vi "2D FFT and IFFT Example.vi"() -> ()   [LabVIEW 2012]
uses:
  Non-User VIs/Error Checking/View Error Log Mode Functional Global.vi
  OpenCLV x64.lvlib
panel:
  out "Labview Data":dbl[][](array[numeric])
  out "OpenCLV Data":dbl[][](array[numeric])
  out "OpenCLV Time":u32
  out "Labview Time":u32
  in  "FFT Dimension":enum16{"1D FFT", "2D FFT"}(ring)=enum."2D FFT"
  in  "Dimension":cluster{"Depth":u64, "Height":u64, "Width":u64}={"Depth"=1, "Height"=1000, "Width"=1024} {"Width" min=1; "Height" min=1; "Depth" min=1}
  # "Outputs"
  # "Inputs - Change before running"
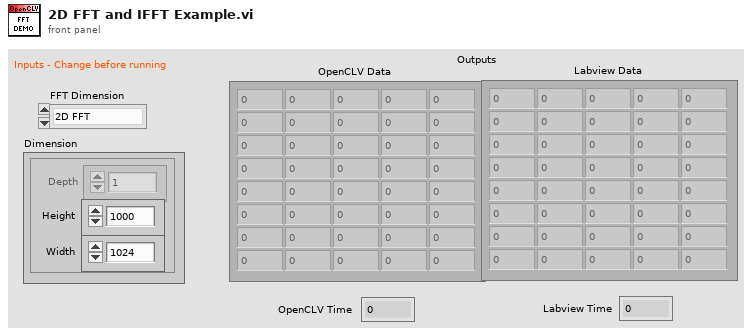
[diagram p1: front panel]
types:
  T1 = enum16{"Allocate", "Compute FFT and IFFT", "Compute Labivew FFT and IFFT", "Clean up"}
  T2 = typedef "OpenCLV x64.lvlib/Device ID.ctl" = u64
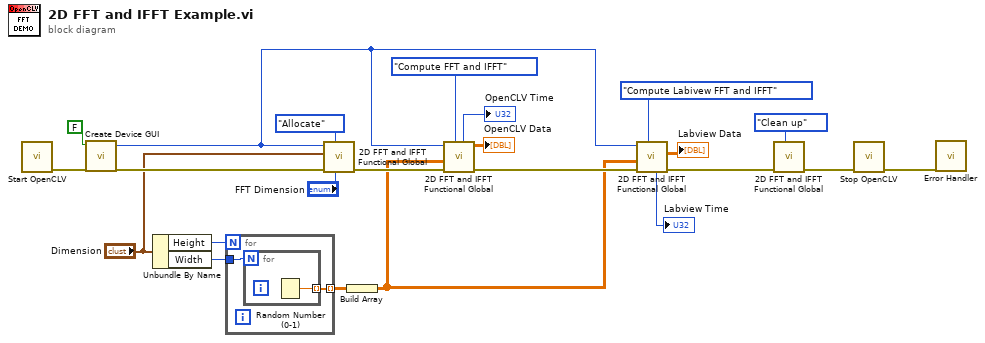
[diagram p0: block diagram]
diagram:
  n1 = call "Start OpenCLV.vi"() -> ("Error Out"=w20:errorcluster)  [unwired: 11 in]
  n2 = call "Create Device GUI.vi"("Error In"=w20, "Skip Configuration"=FALSE) -> ("error constant"=w19:errorcluster, "Device Reference"=w11:T2)  [unwired: 8 in]
  n3 = Unbundle By Name("Dimension") -> ("Height"=w22:u64, "Width"=w21:u64)
  n4 = for {
    N: w22 -> [_]
    tunnel: w21 -> [w25]
    tunnel: [w24] -> w13 mode=indexing
    n5 = for {
      N: w25 -> [_]
      tunnel: [w26] -> w24 mode=indexing
      n6 = Random Number (0-1)() -> (number: 0 to 1=w26:dbl)
    }
  }
  n7 = call "2D FFT and IFFT Functional Global.vi"("FFT Dimension"="FFT Dimension", "FFT States"=T1."Allocate", "Error In"=w19, "Dimension FFT"="Dimension", "Device"=w11) -> ("Error Out"=w14:errorcluster)  [unwired: 2 in, 4 out]
  n8 = Build Array(w13) -> (w10:dbl[][][])
  n9 = call "2D FFT and IFFT Functional Global.vi"("FFT States"=T1."Compute FFT and IFFT", "Error In"=w14, "Real In"=w10, "Device"=w11) -> ("Error Out"=w12:errorcluster, "OpenCLV Data"=→"OpenCLV Data":dbl[][], "OpenCLV Time"=→"OpenCLV Time":u32)  [unwired: 3 in, 2 out]
  n10 = call "2D FFT and IFFT Functional Global.vi"("FFT States"=T1."Compute Labivew FFT and IFFT", "Error In"=w12, "Real In"=w10, "Device"=w11) -> ("Error Out"=w6:errorcluster, "Labview Data"=→"Labview Data":dbl[][], "Labview Time"=→"Labview Time":u32)  [unwired: 3 in, 2 out]
  n11 = call "2D FFT and IFFT Functional Global.vi"("FFT States"=T1."Clean up", "Error In"=w6) -> ("Error Out"=w4:errorcluster)  [unwired: 5 in, 4 out]
  n12 = call "Stop OpenCLV.vi"("Error In"=w4) -> ("Error Out"=w3:errorcluster)  [unwired: 10 in]
  n13 = call-poly "Error Handler.vi"("Error In"=w3) -> ()  [unwired: 10 in, 1 out]
